vi "listen connection LV15.vi"(10 "service name":string="192.168.1.10") -> (2 "Boolean 3":bool, 3 "data out":string)   [LabVIEW 2015]
uses:
  Galobal variable_TI.vi
panel:
  out "String":string
  out "Coordinate 3":string
  out "Numeric 2":i32
  out "error out 3":errorcluster
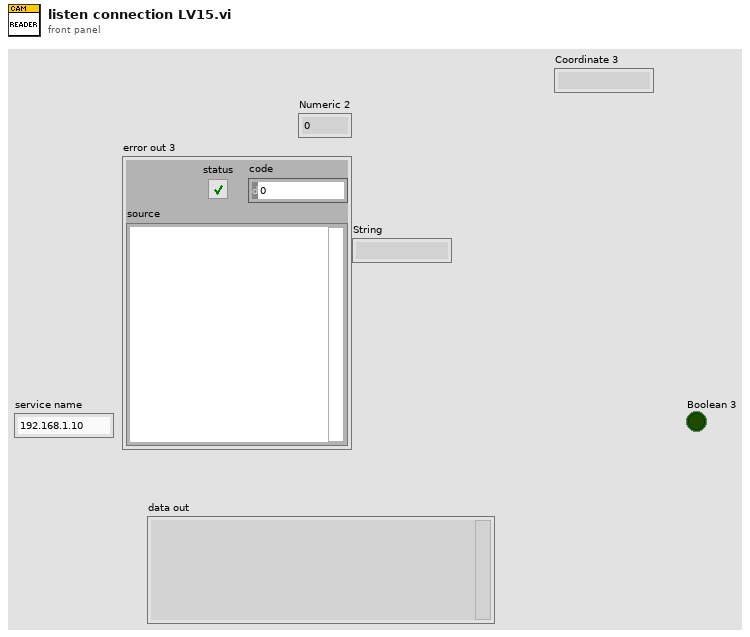
[diagram p1: front panel]
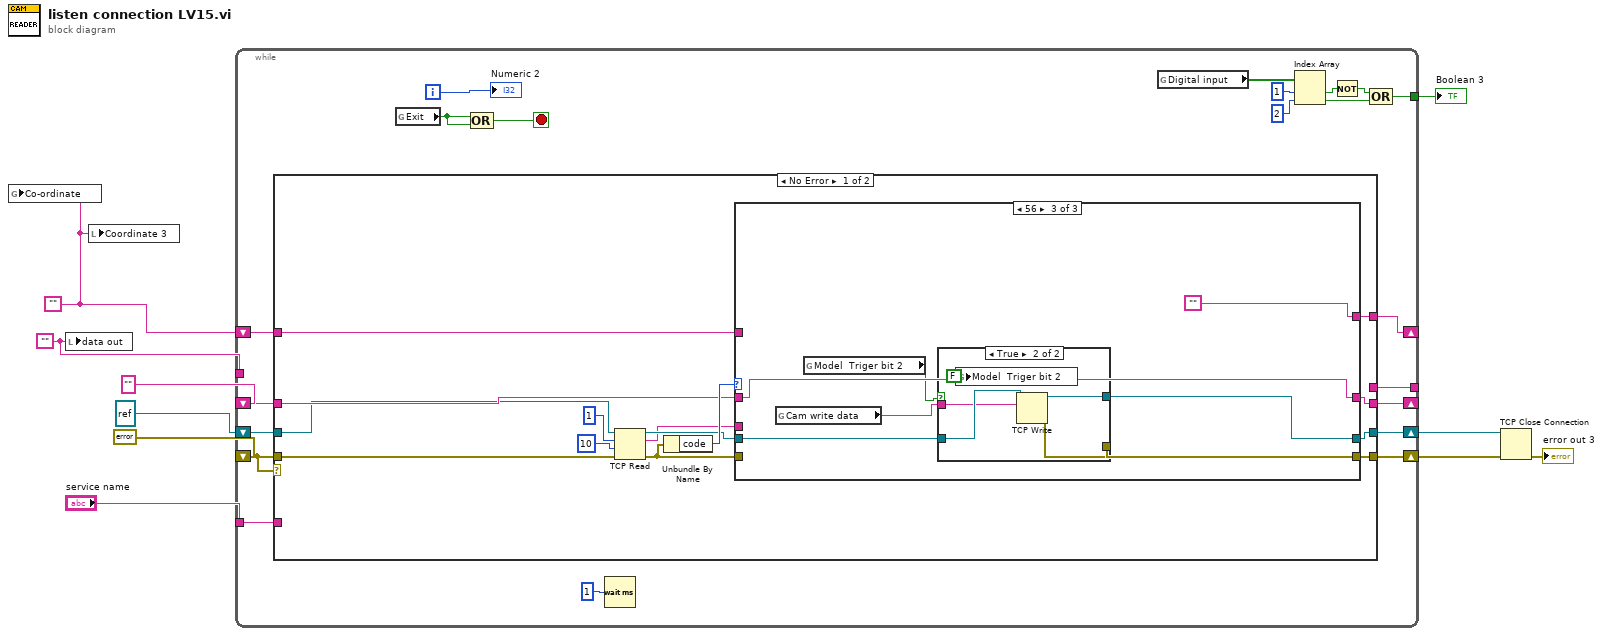
[diagram p0: block diagram]
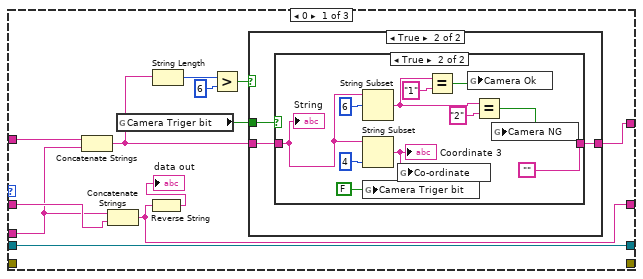
[diagram p2: hidden frame]
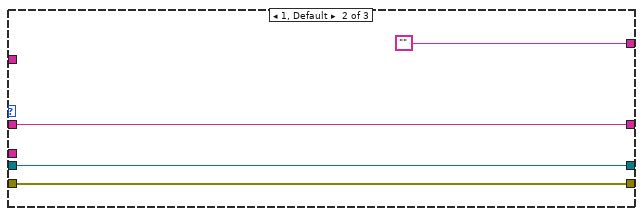
[diagram p5: hidden frame]
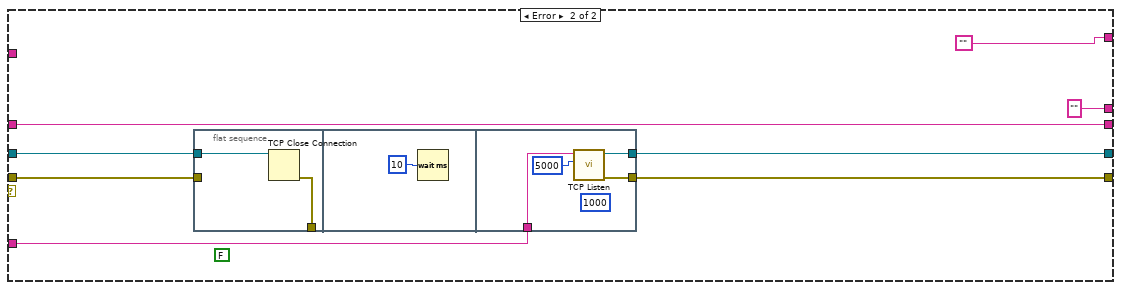
[diagram p7: hidden frame]
diagram:
  w1 = ""
  w2 = ""
  n1 = global write "Galobal variable_TI.vi" "Co-ordinate"(w1) -> ()
  n2 = local write "data out"(w2) -> ()
  n3 = local write "Coordinate 3"(w1) -> ()
  n4 = while {
    tunnel: [w29] -> _
    shift-right: [w31] -> w10
    shift-left: refnum<k5> refnum ("connection ID") -> [w28]
    shift-right: [w30] -> w9
    shift-left: errorcluster {"status"=FALSE, "code"=0, "source"=""} ("error out") -> [w27]
    tunnel: "service name" -> [w26]
    shift-right: [w16] -> _
    shift-left: "" -> [w25]
    tunnel: [w15] -> w3
    tunnel: w2 -> [_]
    shift-right: [w12] -> _
    shift-left: w1 -> [w13]
    i -> [w11]
    stop <- w23 stop-if-true
    n5 = case shown="No Error" w27 {
      tunnel: [w42 w94] -> w31
      tunnel: [w41 w93] -> w30
      tunnel: [_ "" ("data out")] -> w29
      tunnel: w28 -> [w33 w98]
      tunnel: w27 -> [w32 w97]
      tunnel: w26 -> [_ w96]
      tunnel: [w36 w95] -> w16
      tunnel: w25 -> [w38 w95]
      tunnel: w13 -> [w35 _]
      tunnel: [w34 ""] -> w12
      frame No Error {
        n6 = TCP Read(connection ID=w33, bytes to read=1, error in (no error)=w32, 9:10 ("timeout ms (25000)")) -> (connection ID out=w43:refnum<k5>, data out=w39:string, error out=w40:errorcluster)  [unwired: 1 in]
        n7 = Unbundle By Name(w40) -> ("code"=w44:i32)
        n8 = case shown="56" w44 {
          tunnel: w43 -> [w57 w76 w80]
          tunnel: [w57 w76 w82] -> w42
          tunnel: [_ w77 w81] -> w41
          tunnel: w40 -> [_ w77 _]
          tunnel: w39 -> [w48 _ _]
          tunnel: [w50 w75 w84] -> w36
          tunnel: w38 -> [w51 w75 w84]
          tunnel: w35 -> [w49 _ _]
          tunnel: [w47 "" ""] -> w34
          frame 0 {
            n9 = Concatenate Strings(w49, w48) -> (w46:string)
            n10 = Concatenate Strings(w48, w51) -> (w50:string)
            n11 = global read "Galobal variable_TI.vi" "Camera Triger bit"() -> (w54:bool)
            n12 = Reverse String(1:w50) -> (0:→"data out":string)
            n13 = String Length(string=w46) -> (length=w56:i32)
            n14 = Greater?(x=w56, y=6) -> (0:w55:bool)
            n15 = case shown="True" w55 {
              tunnel: w54 -> [_ w61]
              tunnel: w46 -> [w58 w60]
              tunnel: [w58 w59] -> w47
              frame False {
              }
              frame True {
                n16 = case shown="True" w61 {
                  tunnel: w60 -> [w62 w64]
                  tunnel: [w62 ""] -> w59
                  frame False {
                  }
                  frame True {
                    n17 = String Subset(string=w64, offset (0)=6) -> (substring=w67:string)  [unwired: 1 in]
                    n18 = String Subset(string=w64, length (rest)=4 ("length (rest)")) -> (substring=w73:string)  [unwired: 1 in]
                    "Coordinate 3" <- w73
                    n19 = global write "Galobal variable_TI.vi" "Camera Triger bit"(FALSE ("CAMERA TRIGGER")) -> ()
                    n20 = global write "Galobal variable_TI.vi" "Co-ordinate"(w73) -> ()
                    n21 = Equal?(x=w67, y="1") -> (x = y?=w66:bool)
                    n22 = global write "Galobal variable_TI.vi" "Camera Ok"(w66) -> ()
                    n23 = Equal?(x=w67, y="2") -> (x = y?=w65:bool)
                    n24 = global write "Galobal variable_TI.vi" "Camera NG"(w65) -> ()
                    "String" <- w64
                  }
                }
              }
            }
          }
          frame 1, Default {
          }
          frame 56 {
            n25 = global read "Galobal variable_TI.vi" "Cam write data"() -> (w78:string)
            n26 = global read "Galobal variable_TI.vi" "Model  Triger bit 2"() -> (w79:bool)
            n27 = case shown="True" w79 {
              tunnel: [w85 w90] -> w82
              tunnel: [_ w89] -> w81
              tunnel: w80 -> [w85 w88]
              tunnel: w78 -> [_ w86]
              frame False {
              }
              frame True {
                n28 = global write "Galobal variable_TI.vi" "Model  Triger bit 2"(FALSE ("Model triger")) -> ()
                n29 = TCP Write(connection ID=w88, data in=w86) -> (connection ID out=w90:refnum<k5>, error out=w89:errorcluster)  [unwired: 2 in, 1 out]
              }
            }
          }
        }
      }
      frame Error {
        (unwired) FALSE
        n30 = flat-sequence {
          tunnel: w98 -> [w100]
          tunnel: w97 -> [_]
          tunnel: [w99] -> _
          tunnel: w96 -> [w104]
          tunnel: [w103] -> w94
          tunnel: [w102] -> w93
          frame #0 {
            n31 = TCP Close Connection(connection ID=w100) -> (error out=w99:errorcluster)  [unwired: 2 in, 1 out]
          }
          frame #1 {
            n32 = Wait (ms)(milliseconds to wait=u32 10) -> ()  [unwired: 1 out]
          }
          frame #2 {
            (unwired) 1000 ("timeout ms (wait forever: -1)")
            n33 = call <vilib>:"TCP Listen.vi"("port"=u16 5000, "service name"=w104) -> ("error out"=w102:errorcluster, "connection ID"=w103:refnum<k5>)  [unwired: 5 in, 3 out]
          }
        }
      }
    }
    n34 = global read "Galobal variable_TI.vi" "Exit"() -> (w14:bool)
    n35 = Compound Arithmetic op=OR(w14, w14) -> (w23:bool)
    n36 = Wait (ms)(milliseconds to wait=u32 1) -> ()  [unwired: 1 out]
    n37 = global read "Galobal variable_TI.vi" "Digital input"() -> (w22:bool[])
    n38 = Index Array(array=w22, index #1=1 ("index"), index #2=2 ("index")) -> (element #1=w19:bool, element #2=w17:bool)
    n39 = Not(x=w19) -> (.not. x?=w18:bool)
    n40 = Compound Arithmetic op=OR(w18, w17) -> (w15:bool)
    "Numeric 2" <- w11
  }
  "Boolean 3" <- w3
  n41 = TCP Close Connection(connection ID=w10, error in (no error)=w9) -> (error out=→"error out 3":errorcluster)  [unwired: 1 in, 1 out]
